vi "STOMP Tester.vi"() -> ()   [LabVIEW 2017]
uses:
  Typedefs/Type_FrameHeader.ctl
  Typedefs/Type_ServerFrame.ctl
  Typedefs/Type_ServerFrameType.ctl
  STOMP.lvclass
  Typedefs/Type_AckHeader.ctl
panel:
  out "message":T1
  in  "ExitButton":bool
  in  "ConnectButton":bool
  in  "Tab Control":enum32{"Publish", "Subscribe"}(tab)=enum."Subscribe"
  in  "SendButton":bool
  in  "SendHeaders":T3[](array[typedef])=[{"Header"="auto-delete", "Value"="true"}, {"Header"="durable", "Value"="false"}]
  in  "SendDestination":string="/exchange/amq.fanout"
  in  "SendMessage":string
  in  "Subscriptions":i32(listbox)=-1
  in  "SubscribeDestination":string="/exchange/amq.fanout"
  in  "Subscribe":bool
  in  "SubscribeHeaders":T3[](array[typedef])=[{"Header"="auto-delete", "Value"="true"}, {"Header"="durable", "Value"="false"}] caption="Headers"
  in  "port":i32=61613
  in  "hostname":string="localhost"
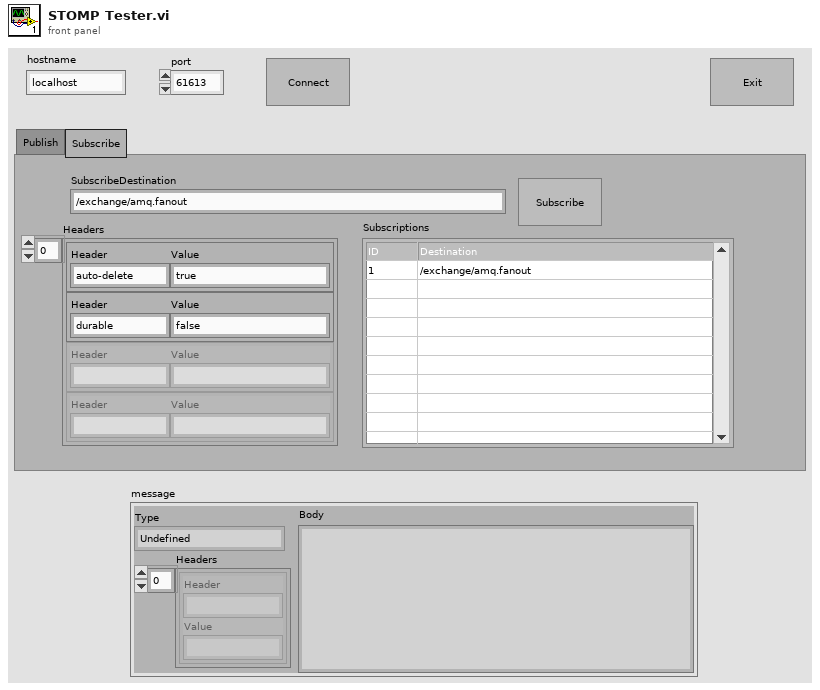
[diagram p1: front panel]
types:
  T1 = typedef "STOMP.lvclass/Type_ServerFrame.ctl" = cluster{"Type":T2, "Headers":cluster{"Header":string, "Value":string}[], "Body":string}
  T2 = typedef "STOMP.lvclass/Type_ServerFrameType.ctl" = enum16{"Undefined", "MESSAGE", "CONNECTED", "RECEIPT", "ERROR"}
  T3 = typedef "STOMP.lvclass/Type_FrameHeader.ctl" = cluster{"Header":string, "Value":string}
  T4 = typedef "STOMP.lvclass/Type_AckHeader.ctl" = enum16{"auto", "client", "client-individual"}
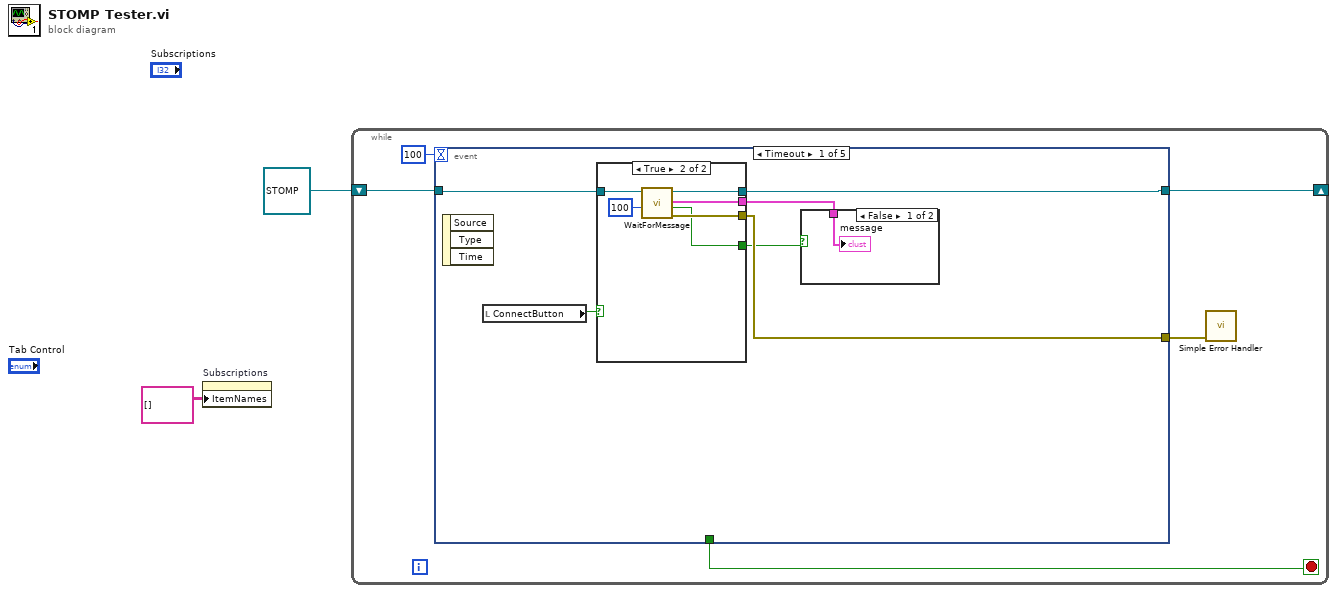
[diagram p0: block diagram]
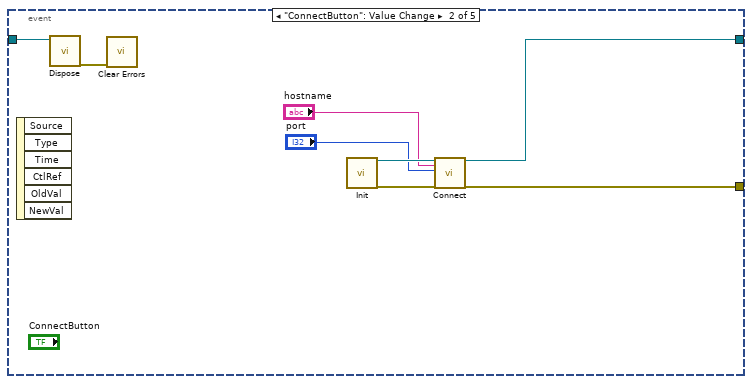
[diagram p4: hidden frame]
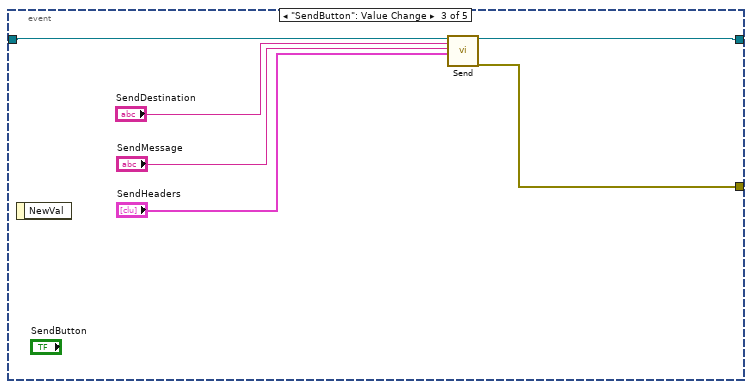
[diagram p5: hidden frame]
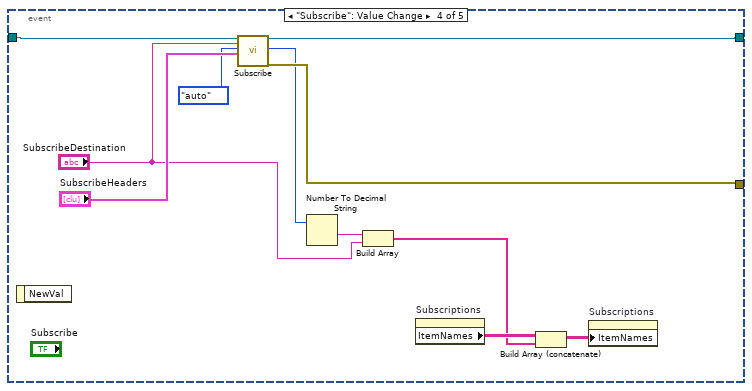
[diagram p6: hidden frame]
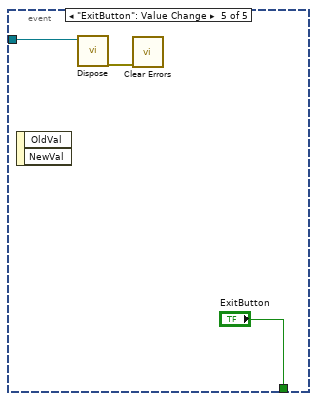
[diagram p7: hidden frame]
diagram:
  n1 = property on="Subscriptions" class="MCListbox (strict)"("ItemNames"=string[][] [] ("Item Names")) -> ()  [unwired: 2 in, 2 out]
  n2 = while {
    shift-right: [w5] -> _
    shift-left: refnum<class "STOMP.lvclass"> refnum ("STOMP in") -> [w6]
    stop <- w7 stop-if-true
    n3 = event shown="[0] Timeout" {
      selector: _ -> [_ _ _ _ _]
      dyn-events: _ -> [_ _ _ _ _]
      timeout: 100 -> [_ _ _ _ _]
      tunnel: [_ _ _ _ "ExitButton"] -> w7
      tunnel: w6 -> [w11 w23 w35 w46 w48]
      tunnel: [w13 w25 w34 w45 _] -> w5
      tunnel: [w12 w24 w30 w42 _] -> w4
      event Timeout {
        n4 = event-data() -> ()  [unwired: 1 in, 3 out]
        n5 = local read "ConnectButton"() -> (w10:bool)
        n6 = case shown="True" w10 {
          tunnel: [w15 w21] -> w13
          tunnel: [_ w20] -> w12
          tunnel: w11 -> [w15 w18]
          tunnel: [_ w17] -> w9
          tunnel: [_ w16] -> w8
          frame False {
          }
          frame True {
            n7 = call-dynamic "WaitForMessage.vi"("timeout in ms (10000)"=100, "STOMP in"=w18) -> ("error out"=w20:errorcluster, "timed out?"=w16:bool, "message"=w17:T1, "STOMP out"=w21:refnum<class "STOMP.lvclass">)  [unwired: 6 in]
          }
        }
        n8 = case shown="False" w8 {
          tunnel: w9 -> [w14 _]
          frame False {
            "message" <- w14
          }
          frame True {
          }
        }
      }
      event "ConnectButton": Value Change {
        n9 = event-data() -> ()  [unwired: 1 in, 6 out]
        n10 = call-dynamic "Dispose.vi"("STOMP in"=w23) -> ("error out"=w22:errorcluster)  [unwired: 9 in, 1 out]
        n11 = call <vilib>:"Clear Errors.vi"("error in (no error)"=w22) -> ()  [unwired: 5 in, 2 out]
        n12 = call "Init.vi"() -> ("STOMP out"=w29:refnum<class "STOMP.lvclass">, "error out"=w28:errorcluster)  [unwired: 18 in]
        n13 = call "Connect.vi"("STOMP in"=w29, "address"="hostname", "port"="port", "error in"=w28) -> ("STOMP out"=w25:refnum<class "STOMP.lvclass">, "error out"=w24:errorcluster)  [unwired: 14 in]
      }
      event "SendButton": Value Change {
        n14 = event-data() -> ()  [unwired: 1 in, 1 out]
        n15 = call-dynamic "Send.vi"("STOMP in"=w35, "Destination"="SendDestination", "Body"="SendMessage", "headers"="SendHeaders") -> ("STOMP out"=w34:refnum<class "STOMP.lvclass">, "error out"=w30:errorcluster)  [unwired: 14 in]
      }
      event "Subscribe": Value Change {
        n16 = event-data() -> ()  [unwired: 1 in, 1 out]
        n17 = call-dynamic "Subscribe.vi"("STOMP in"=w46, "Destination"="SubscribeDestination", "ack"=Type_AckHeader."auto", "headers"="SubscribeHeaders") -> ("STOMP out"=w45:refnum<class "STOMP.lvclass">, "Subscription ID"=w38:u64, "error out"=w42:errorcluster)  [unwired: 13 in]
        n18 = Number To Decimal String(number=w38) -> (decimal integer string=w39:string)  [unwired: 1 in]
        n19 = Build Array(w39, "SubscribeDestination") -> (w36:string[])
        n20 = property on="Subscriptions" class="MCListbox (strict)"() -> ("ItemNames"=w41:string[][])  [unwired: 2 in, 2 out]
        n21 = Build Array (concatenate)(w41, w36) -> (w40:string[][])
        n22 = property on="Subscriptions" class="MCListbox (strict)"("ItemNames"=w40) -> ()  [unwired: 2 in, 2 out]
      }
      event "ExitButton": Value Change {
        n23 = event-data() -> ()  [unwired: 1 in, 2 out]
        n24 = call-dynamic "Dispose.vi"("STOMP in"=w48) -> ("error out"=w47:errorcluster)  [unwired: 9 in, 1 out]
        n25 = call <vilib>:"Clear Errors.vi"("error in (no error)"=w47) -> ()  [unwired: 5 in, 2 out]
      }
    }
    n26 = call <vilib>:"Simple Error Handler.vi"("error in (no error)"=w4) -> ()  [unwired: 4 in, 5 out]
  }
